vi "CH2 ON (SubVI).vi"() -> (3 "String":string)   [LabVIEW 2018]
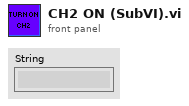
[diagram p1: front panel]
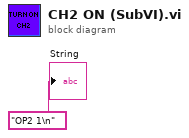
[diagram p0: block diagram]
diagram:
  "String" <- "OP2 1\n"
